vi "Autonomia v1.vi"(8 "Autonomia ?":bool, 11 "Ster Wej":cluster{dbl, dbl}) -> (3 "Ster Wyj":cluster{dbl, dbl})   [LabVIEW 2014]
panel:
  out "P 7":dbl(slide) scale=-66000.0..66000.0
  out "P 6":dbl(slide) scale=-66000.0..66000.0
  out "L 7":dbl(slide) scale=-66000.0..66000.0
  out "L 6":dbl(slide) scale=-66000.0..66000.0
  out "wyj pred":cluster{u16, u16, u16, u16, u16, u16} {"?" scale=0.0..65000.0; "?" scale=0.0..65000.0; "?" scale=0.0..65000.0; "?" scale=0.0..65000.0; "?" scale=0.0..65000.0; "?" scale=0.0..65000.0}
  out "L 5":dbl(slide) scale=-66000.0..66000.0
  out "P 5":dbl(slide) scale=-66000.0..66000.0
  in  "Time Stamp":timestamp
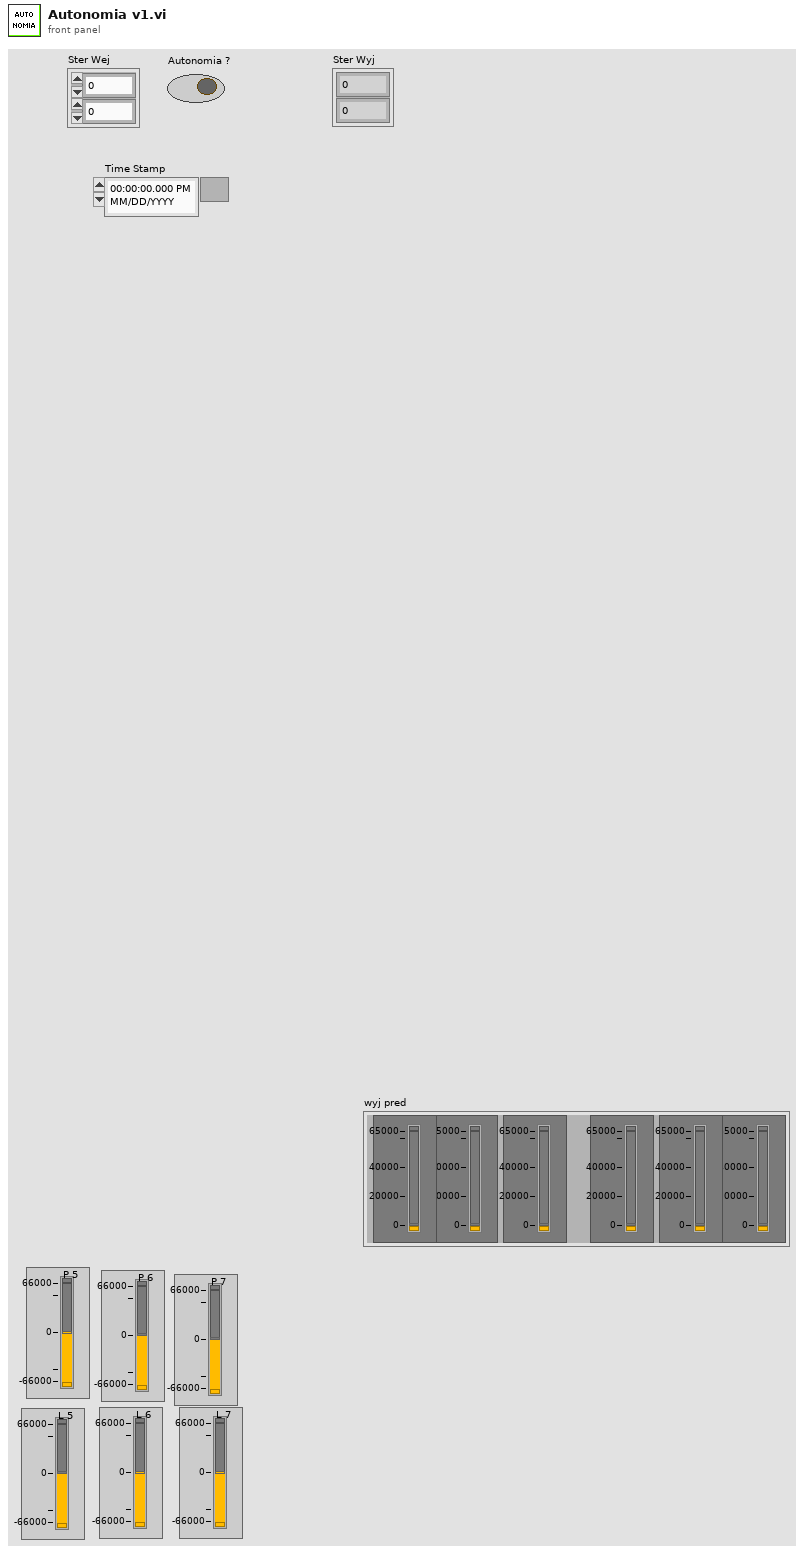
[diagram p1: front panel]
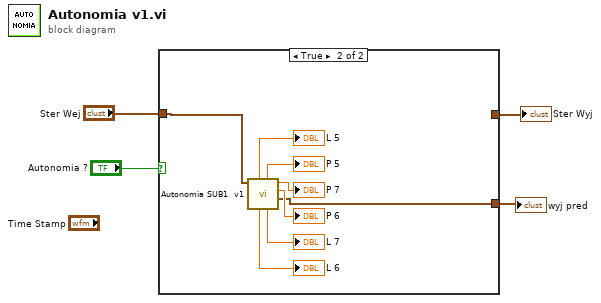
[diagram p0: block diagram]
diagram:
  n1 = case shown="True" "Autonomia ?" {
    tunnel: "Ster Wej" -> [w5 w7]
    tunnel: [w5 _] -> w3
    tunnel: [_ w6] -> w1
    frame False {
    }
    frame True {
      n2 = call "Autonomia SUB1  v1.vi"("Ster Wej"=w7) -> ("wyj pred"=w6:cluster{u16, u16, u16, u16, u16, u16}, "P 6"=→"P 6":dbl, "P 7"=→"P 7":dbl, "L 7"=→"L 7":dbl, "P 5"=→"P 5":dbl, "L 6"=→"L 6":dbl, "L 5"=→"L 5":dbl)  [unwired: 4 in]
    }
  }
  "Ster Wyj" <- w3
  "wyj pred" <- w1
